vi "DB_Action.vi"(8 "error in":errorcluster, 10 "Command Text":string="select max(ID) from UUT_RESULT;", 11 "路径":path=path "E:/3_PC_Module Tool/FCT_4_CommonVI/23_LabviewTester/0_Tester/0_plugins/Plugin_DB/Sub/DB_Report2014.mdb") -> (0 "error out":errorcluster, 2 "Data":string[][](array[string]))   [LabVIEW 2015, in "Settings-Style.lvlib"]
uses:
  Settings-Style.lvlib
  <vilib>/addons/database/Connection.llb/Conn ObjectReference.ctl
  <vilib>/addons/database/Connection.llb/DB Tools Open Connec (String).vi
  <vilib>/addons/database/Connection.llb/Conn Execute.vi
  <vilib>/addons/database/Recordset.llb/Rec Fetch Recordset Data (R).vi
  <vilib>/addons/database/Recordset.llb/Rec Destroy - Connection.vi
  <vilib>/addons/database/_DB Variant To Data/Database Variant To Data.xnode
  <vilib>/addons/database/NI_Database_API.lvlib
panel:
  # "SELECT  UUT_RESULT.* FROM UUT_RESULT,STEP_RESULT,UUT_STEP_STATUS,UUT_STEP_VALUE WHERE  START_DATE_TIME>=#2014/04/09 10:15:47# AND START_DATE_TIME<=#2014/05/09 10:15:47#  AND UUT_RESULT.ID = UUT_STEP_STATUS.UUT_RESULT  and UUT_RESULT.ID >=100;"
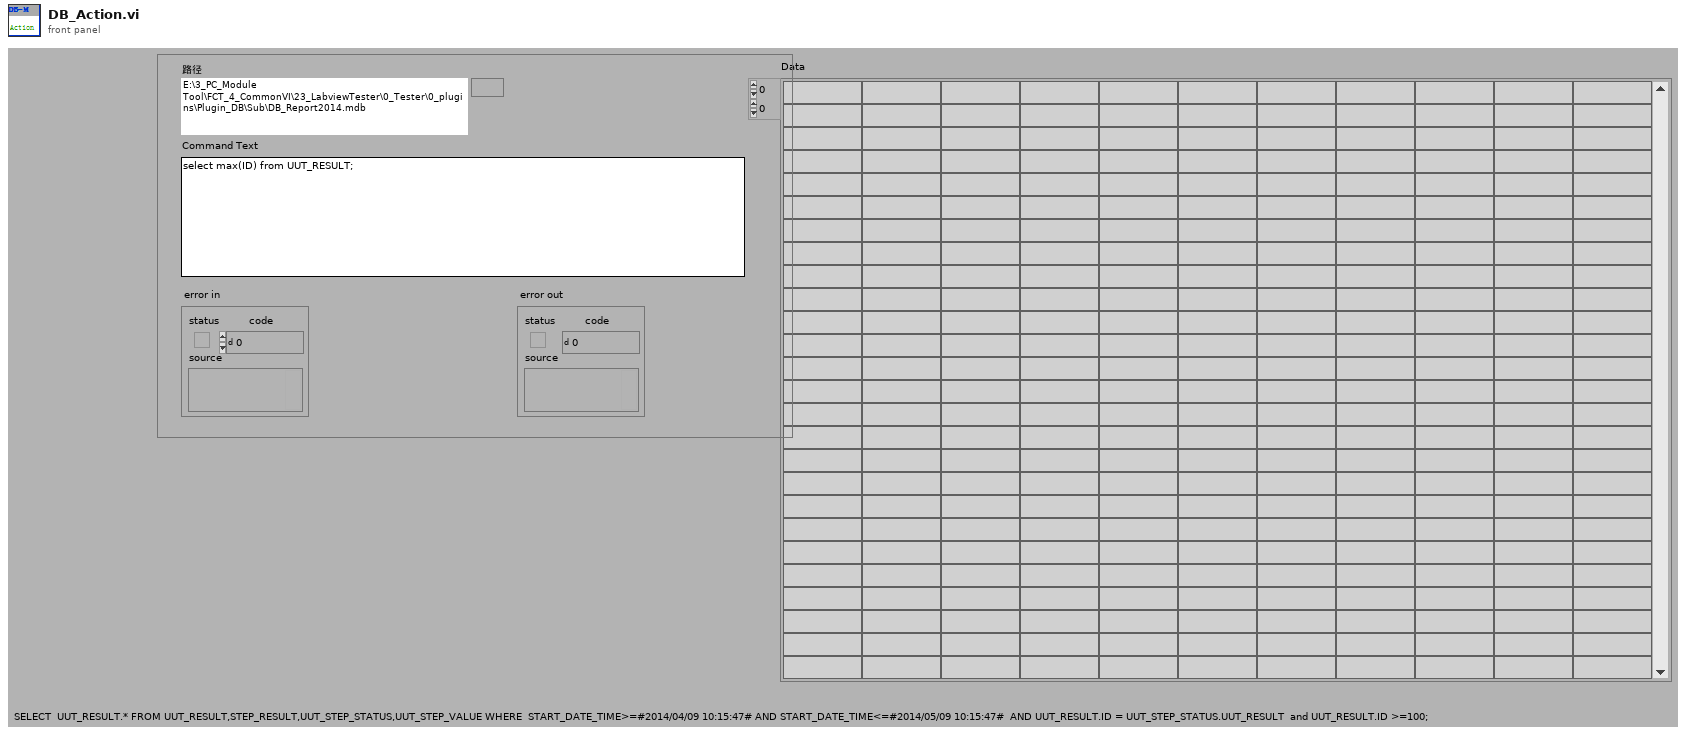
[diagram p1: front panel]
types:
  T1 = typedef "NI_Database_API.lvlib/Conn ObjectReference.ctl" = refnum<k1>
  T2 = typedef "NI_Database_API.lvlib/Rec ObjectReference.ctl" = refnum<k1>
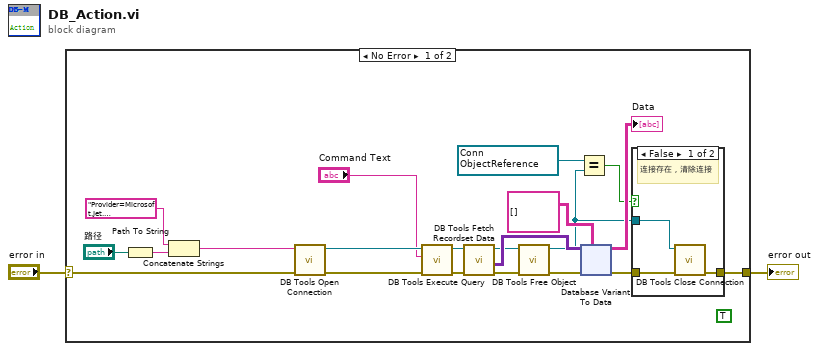
[diagram p0: block diagram]
diagram:
  n1 = case shown="No Error" "error in" {
    selector: "error in" -> [w22 w72]
    tunnel: [w23 w72] -> w2
    frame No Error {
      w17 = T1 refnum items=["Connection"] ("connection reference")
      (unwired) TRUE
      n2 = Path To String(path="路径") -> (string=w19:string)
      n3 = Concatenate Strings("Provider=Microsoft.Jet.OLEDB.4.0;Data Source=" ("ConnectionString"), w19) -> (w18:string)
      n4 = call-poly <vilib>:"DB Tools Open Connection.vi"("error in (no error)"=w22, "connection information"=w18) -> ("error out"=w16:errorcluster, "connection reference"=w15:T1)  [unwired: 6 in]
      n5 = call-poly <vilib>:"DB Tools Execute Query.vi"("error in (no error)"=w16, "SQL query"="Command Text", "connection reference"=w15) -> ("error out"=w12:errorcluster, "recordset reference"=w13:T2)  [unwired: 5 in]
      n6 = call-poly <vilib>:"DB Tools Fetch Recordset Data.vi"("error in (no error)"=w12, "recordset reference"=w13) -> ("error out"=w7:errorcluster, "recordset data"=w11:variant[][], "recordset reference out"=w8:T2)  [unwired: 3 in]
      n7 = call-poly <vilib>:"DB Tools Free Object.vi"("error in (no error)"=w7, "recordset reference"=w8) -> ("error out"=w6:errorcluster, "connection reference"=w3:T1)  [unwired: 8 in]
      n8 = Equal?(x=w17, y=w3) -> (x = y?=w4:bool)
      n9 = xnode "Database Variant To Data"("database variant"=w11, "error in (no error)"=w6, "type"=string[][] [] ("Data")) -> ("data"=→"Data":string[][], "error out"=w5:errorcluster)
      n10 = case shown="False" w4 {
        tunnel: [w26 w27] -> w23
        tunnel: w5 -> [w25 w27]
        tunnel: w3 -> [w24 _]
        frame False {
          # "连接存在，清除连接"
          n11 = call <vilib>:"DB Tools Close Connection.vi"("error in (no error)"=w25, "connection reference"=w24) -> ("error out"=w26:errorcluster)  [unwired: 5 in]
        }
        frame True {
          # "连接为空，不操作。"
        }
      }
    }
    frame Error {
    }
  }
  "error out" <- w2
